vi "WPI_ADI_IMU_Open.vi"(8 "error in":errorcluster, 9 "AHRS Algorithm":enum16{"Complementary", "Madgwick"}(ring), 10 "Yaw Axis":enum16{"X", "Y", "Z"}(ring)=enum."Z", 11 "SPI Chip Select":T3=enum."SPI MXP") -> (0 "error out":errorcluster, 3 "ADI IMU Interrupt DevRef":T1={"SimpleGyroDevRef"={"DevStatus"={"status"=FALSE, "code"=0, "source"=""}, "Handle"=0, "SPI Bus"=enum."SPI On-Board, CS0", "Device Found"=FALSE, "Sample Rate"=0.0, "Device Ready"=FALSE, "Yaw Axis"=enum."Z", "AHRS Algorithm"=enum."Complementary"}, "InterruptRef"={"DevStatus"={"status"=FALSE, "code"=0, "source"=""}, "InterruptIndex"=enum."0"}} {"SimpleGyroDevRef"."Sample Rate" min=0.25 max=100.0 step=0.25})   [LabVIEW 2015, in "FRC ADI MXP IMU.lvlib"]
doc: "Initiates communication between an Analog Devices MXP IMU and the RoboRIO."
uses:
  FRC ADI MXP IMU.lvlib
  <vilib>/Rock Robotics/SystemInterfaces/spilib/spi_bus.ctl
  WPI_AnalogDevicesIMUInterruptDevRef.ctl
  WPI_AnalogDevicesIMUDevRef.ctl
  <vilib>/Rock Robotics/WPI/Interrupt/WPI_InterruptRef.ctl
  <vilib>/Rock Robotics/SystemInterfaces/Interrupt/FPGA_InterruptIndex.ctl
  <vilib>/Rock Robotics/WPI/SPI/WPI_SPIMode.ctl
  <vilib>/Rock Robotics/SystemInterfaces/DIO/FPGA_DIOChannel.ctl
  WPI_IMU_ADIS16448_Registers.ctl
  <vilib>/Rock Robotics/WPI/Counter/WPI_CounterDigitalInputToDigitalSource.vi
  <vilib>/Rock Robotics/SystemInterfaces/CounterEncoderSourceConvertion/FPGA_CounterEncoderSourceConvertionLVSourceTypeToFPGAType.vi
  <vilib>/Rock Robotics/WPI/Interrupt/WPI_InterruptCache.vi
  <vilib>/Rock Robotics/SystemInterfaces/Interrupt/FPGA_InterruptWriteConfiguration.vi
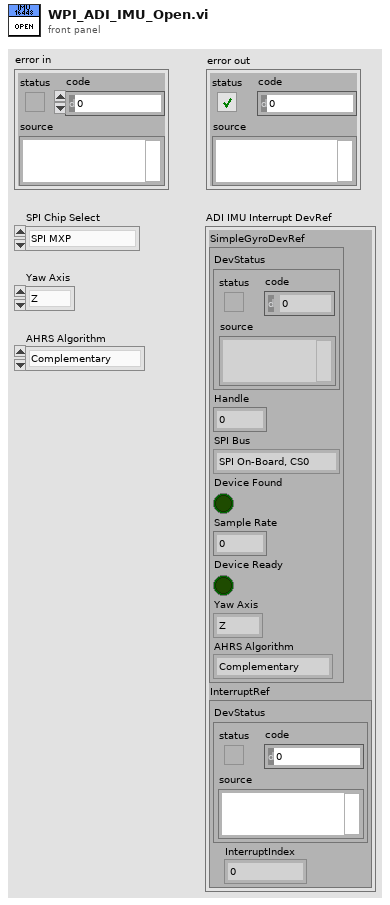
[diagram p1: front panel]
types:
  T1 = typedef "FRC ADI MXP IMU.lvlib/WPI_AnalogDevicesIMUInterruptDevRef.ctl" = cluster{"SimpleGyroDevRef":T2, "InterruptRef":T4}
  T2 = typedef "FRC ADI MXP IMU.lvlib/WPI_AnalogDevicesIMUDevRef.ctl" = cluster{"DevStatus":errorcluster, "Handle":i32, "SPI Bus":T3, "Device Found":bool, "Sample Rate":dbl, "Device Ready":bool, "Yaw Axis":enum16{"X", "Y", "Z"}, "AHRS Algorithm":enum16{"Complementary", "Madgwick"}}
  T3 = typedef "spi_bus.ctl" = enum16{"SPI On-Board, CS0", "SPI On-Board, CS1", "SPI On-Board, CS2", "SPI On-Board, CS3", "SPI MXP", "Invalid"}
  T4 = typedef "WPI_InterruptRef.ctl" = cluster{"DevStatus":errorcluster, "InterruptIndex":T5}
  T5 = typedef "FPGA_InterruptIndex.ctl" = enum8{"0", "1", "2", "3", "4", "5", "6", "7", "Invalid"}
  T6 = typedef "FPGA_DIOChannel.ctl" = enum8{"DIO 0", "DIO 1", "DIO 2", "DIO 3", "DIO 4", "DIO 5", "DIO 6", "DIO 7", "DIO 8", "DIO 9", "DIO MXP 0", "DIO MXP 1", "DIO MXP 2", "DIO MXP 3", "DIO MXP 4", "DIO MXP 5", "DIO MXP 6", "DIO MXP 7", "DIO MXP 8", "DIO MXP 9", "DIO MXP 10", "DIO MXP 11", "DIO MXP 12", "DIO MXP 13", "DIO MXP 14", "DIO MXP 15", "Invalid"}
  T7 = typedef "WPI_SPIMode.ctl" = enum16{"Mode 0 (Clk Idle Low,Sample on Leading)", "Mode 1 (Clk Idle Low,Sample on Trailing)", "Mode 2 (Clk Idle High,Sample on Leading)", "Mode 3 (Clk Idle High,Sample on Trailing)"}
  T8 = typedef "FRC ADI MXP IMU.lvlib/WPI_IMU_ADIS16448_Registers.ctl" = u8
  T9 = typedef "WPI_DigitalOutputDevRef.ctl" = cluster{"DIO Channel":T6, "DevStatus":errorcluster}
  T10 = typedef "WPI_SPIDevRef.ctl" = cluster{"DevStatus":errorcluster, "Handle":i32, "SPI Bus":T3}
  T11 = typedef "WPI_DigitalInputDevRef.ctl" = cluster{"DevStatus":errorcluster, "DIO Channel":T6}
  T12 = typedef "FPGA_CounterEncoderSourceConvertionLVSourceType.ctl" = cluster{"DevStatus":errorcluster, "AnalogTriggerMode?":bool, "DigitalMode":cluster{"DIO Channel":T13}, "AnalogTriggerMode":cluster{"AnalogTriggerIndex":T14, "OutputType":T15}}
  T13 = typedef "FPGA_DIODigitalSourceChannel.ctl" = enum8{"DIO 0", "DIO 1", "DIO 2", "DIO 3", "DIO 4", "DIO 5", "DIO 6", "DIO 7", "DIO 8", "DIO 9", "DIO MXP 0", "DIO MXP 1", "DIO MXP 2", "DIO MXP 3", "DIO MXP 4", "DIO MXP 5", "DIO MXP 6", "DIO MXP 7", "DIO MXP 8", "DIO MXP 9", "DIO MXP 10", "DIO MXP 11", "DIO MXP 12", "DIO MXP 13", "DIO MXP 14", "DIO MXP 15", "Disabled"}
  T14 = typedef "FPGA_AnalogTriggerIndex.ctl" = enum8{"Trig 0", "Trig 1", "Trig 2", "Trig 3", "Trig 4", "Trig 5", "Trig 6", "Trig 7", "Invalid"}
  T15 = typedef "FPGA_AnalogTriggerOutType.ctl" = enum16{"InWindow", "TriggerState", "Rising", "Falling"}
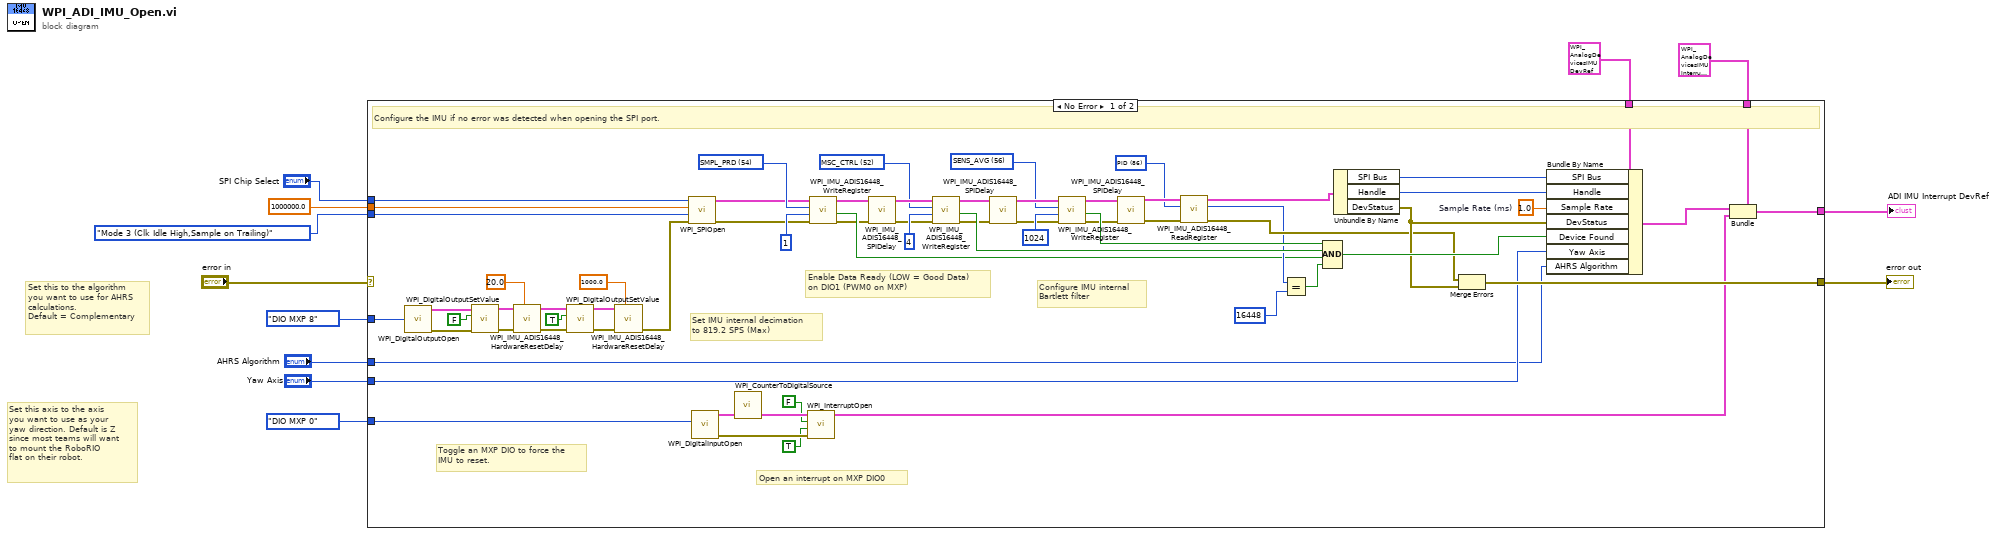
[diagram p0: block diagram]
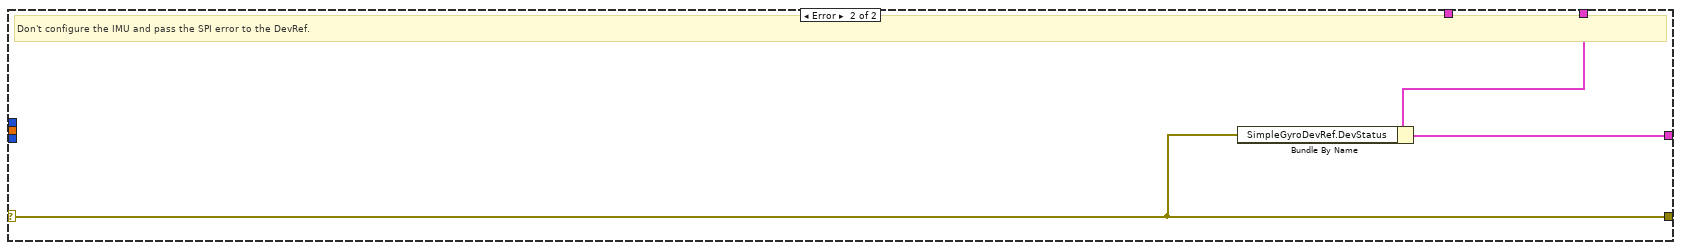
[diagram p2: hidden frame]
diagram:
  # "Set this to the algorithm\nyou want to use for AHRS\ncalculations. \nDefault = Complementary"
  # "Set this axis to the axis\nyou want to use as your\nyaw direction. Default is Z\nsince most teams will want \nto mount the RoboRIO\nflat on their robot."
  n1 = case shown="No Error" "error in" {
    selector: "error in" -> [_ w79]
    tunnel: "SPI Chip Select" -> [w77 _]
    tunnel: 1000000.0 ("Clock Rate (Hz)") -> [w76 _]
    tunnel: WPI_SPIMode."Mode 3 (Clk Idle High,Sample on Trailing)" ("Mode (3)") -> [w75 _]
    tunnel: [w66 w79] -> w8
    tunnel: T2 {"DevStatus"={"status"=FALSE, "code"=0, "source"=""}, "Handle"=0, "SPI Bus"=enum."SPI On-Board, CS0", "Device Found"=FALSE, "Sample Rate"=0.0, "Device Ready"=FALSE, "Yaw Axis"=enum."Z", "AHRS Algorithm"=enum."Complementary"} ("SimpleGyroDevRef 2") -> [w74 _]
    tunnel: [w56 w78] -> w1
    tunnel: T1 {"SimpleGyroDevRef"={"DevStatus"={"status"=FALSE, "code"=0, "source"=""}, "Handle"=0, "SPI Bus"=enum."SPI On-Board, CS0", "Device Found"=FALSE, "Sample Rate"=0.0, "Device Ready"=FALSE, "Yaw Axis"=enum."Z", "AHRS Algorithm"=enum."Complementary"}, "InterruptRef"={"DevStatus"={"status"=FALSE, "code"=0, "source"=""}, "InterruptIndex"=enum."0"}} ("output cluster") -> [w55 w80]
    tunnel: FPGA_DIOChannel."DIO MXP 0" ("DIO Channel") -> [w54 _]
    tunnel: "Yaw Axis" -> [w47 _]
    tunnel: "AHRS Algorithm" -> [w46 _]
    tunnel: FPGA_DIOChannel."DIO MXP 8" ("DIO Channel") -> [w16 _]
    frame No Error {
      w30 = T8 54 items=["GLOB_CMD"=62, "SEQ_CNT"=58, "SMPL_PRD"=54, "SENS_AVG"=56, "MSC_CTRL"=52, "ERROR_FLAGS"=60, "TEMP"=44, "BARO"=40, "Z_MAG"=36, "Y_MAG"=32, "X_MAG"=28, "Z_ACCEL"=24, "Y_ACCEL"=20, "X_ACCEL"=16, "Z_GYRO"=12, "Y_GYRO"=8, "X_GYRO"=4, "PID"=86] ("ADIS16448 Register")
      w31 = T8 52 items=["GLOB_CMD"=62, "SEQ_CNT"=58, "SMPL_PRD"=54, "SENS_AVG"=56, "MSC_CTRL"=52, "ERROR_FLAGS"=60, "TEMP"=44, "BARO"=40, "Z_MAG"=36, "Y_MAG"=32, "X_MAG"=28, "Z_ACCEL"=24, "Y_ACCEL"=20, "X_ACCEL"=16, "Z_GYRO"=12, "Y_GYRO"=8, "X_GYRO"=4, "PID"=86] ("ADIS16448 Register")
      w32 = T8 56 items=["GLOB_CMD"=62, "SEQ_CNT"=58, "SMPL_PRD"=54, "SENS_AVG"=56, "MSC_CTRL"=52, "ERROR_FLAGS"=60, "TEMP"=44, "BARO"=40, "Z_MAG"=36, "Y_MAG"=32, "X_MAG"=28, "Z_ACCEL"=24, "Y_ACCEL"=20, "X_ACCEL"=16, "Z_GYRO"=12, "Y_GYRO"=8, "X_GYRO"=4, "PID"=86] ("ADIS16448 Register")
      w33 = T8 86 items=["GLOB_CMD"=62, "SEQ_CNT"=58, "SMPL_PRD"=54, "SENS_AVG"=56, "MSC_CTRL"=52, "ERROR_FLAGS"=60, "TEMP"=44, "BARO"=40, "Z_MAG"=36, "Y_MAG"=32, "X_MAG"=28, "Z_ACCEL"=24, "Y_ACCEL"=20, "X_ACCEL"=16, "Z_GYRO"=12, "Y_GYRO"=8, "X_GYRO"=4, "PID"=86] ("ADIS16448 Register")
      w71 = 1.0  # Sample Rate (ms)
      # "Toggle an MXP DIO to force the\nIMU to reset."
      # "Open an interrupt on MXP DIO0"
      # "Configure IMU internal\nBartlett filter"
      # "Enable Data Ready (LOW = Good Data) \non DIO1 (PWM0 on MXP)"
      # "Set IMU internal decimation\nto 819.2 SPS (Max)"
      # "Configure the IMU if no error was detected when opening the SPI port."
      n2 = call <vilib>:"WPI_DigitalOutputOpen.vi"("DIO Channel"=w16) -> ("error out"=w26:errorcluster, "DigitalOutputDevRef"=w27:T9)  [unwired: 9 in]
      n3 = call <vilib>:"WPI_DigitalOutputSetValue.vi"("error in (no error)"=w26, "Value"=FALSE, "DigitalOutputDevRef"=w27) -> ("error out"=w24:errorcluster, "DigitalOutputDevRef"=w25:T9)  [unwired: 7 in]
      n4 = call "WPI_IMU_ADIS16448_HardwareResetDelay.vi"("Delay (ms)"=20.0, "error in"=w24, "DigitalOutputDevRef"=w25) -> ("error out"=w23:errorcluster, "DigitalOutputDevRef"=w22:T9)  [unwired: 7 in]
      n5 = call <vilib>:"WPI_DigitalOutputSetValue.vi"("error in (no error)"=w23, "Value"=TRUE, "DigitalOutputDevRef"=w22) -> ("error out"=w20:errorcluster, "DigitalOutputDevRef"=w19:T9)  [unwired: 7 in]
      n6 = call "WPI_IMU_ADIS16448_HardwareResetDelay.vi"("Delay (ms)"=1000.0, "error in"=w20, "DigitalOutputDevRef"=w19) -> ("error out"=w15:errorcluster)  [unwired: 7 in, 1 out]
      n7 = call <vilib>:"WPI_SPIOpen.vi"("error in"=w15, "Mode (3)"=w75, "Clock Rate (Hz)"=w76, "SPI Bus"=w77) -> ("error out"=w13:errorcluster, "SPIDevRef"=w14:T10)  [unwired: 6 in]
      n8 = call <vilib>:"WPI_DigitalInputOpen.vi"("DIO Channel"=w54) -> ("error out"=w61:errorcluster, "DigitalInputDevRef"=w63:T11)  [unwired: 9 in]
      n9 = call-poly <vilib>:"WPI_CounterToDigitalSource.vi"("DigitalInputDevRef"=w63) -> ("Digital Source"=w62:T12)  [unwired: 6 in]
      n10 = call <vilib>:"WPI_InterruptOpen.vi"("error in (no error)"=w61, "Falling Edge"=TRUE, "Rising Edge"=FALSE, "Source"=w62) -> ("InterruptRef"=w58:T4)  [unwired: 6 in, 1 out]
      n11 = call "WPI_IMU_ADIS16448_WriteRegister.vi"("error in (no error)"=w13, "Data"=u16 1, "ADIS16448 Register"=w30, "SPIDevRef in"=w14) -> ("error out"=w44:errorcluster, "Write OK?"=w48:bool, "SPIDevRef out"=w45:T10)  [unwired: 4 in, 1 out]
      n12 = call "WPI_IMU_ADIS16448_SPIDelay.vi"("error in"=w44, "SPIDevRef in"=w45) -> ("error out"=w42:errorcluster, "SPIDevRef out"=w43:T10)  [unwired: 8 in]
      n13 = call "WPI_IMU_ADIS16448_WriteRegister.vi"("error in (no error)"=w42, "Data"=u16 4, "ADIS16448 Register"=w31, "SPIDevRef in"=w43) -> ("error out"=w40:errorcluster, "Write OK?"=w68:bool, "SPIDevRef out"=w41:T10)  [unwired: 4 in, 1 out]
      n14 = call "WPI_IMU_ADIS16448_SPIDelay.vi"("error in"=w40, "SPIDevRef in"=w41) -> ("error out"=w39:errorcluster, "SPIDevRef out"=w38:T10)  [unwired: 8 in]
      n15 = call "WPI_IMU_ADIS16448_WriteRegister.vi"("error in (no error)"=w39, "Data"=u16 1024, "ADIS16448 Register"=w32, "SPIDevRef in"=w38) -> ("error out"=w36:errorcluster, "Write OK?"=w64:bool, "SPIDevRef out"=w37:T10)  [unwired: 4 in, 1 out]
      n16 = call "WPI_IMU_ADIS16448_SPIDelay.vi"("error in"=w36, "SPIDevRef in"=w37) -> ("error out"=w34:errorcluster, "SPIDevRef out"=w35:T10)  [unwired: 8 in]
      n17 = call "WPI_IMU_ADIS16448_ReadRegister.vi"("error in (no error)"=w34, "ADIS16448 Register"=w33, "SPIDevRef in"=w35) -> ("error out"=w52:errorcluster, "Register Value"=w51:u16, "SPIDevRef out"=w53:T10)  [unwired: 6 in]
      n18 = Equal?(x=w51, y=u16 16448) -> (x = y?=w29:bool)
      n19 = Compound Arithmetic op=AND(w64, w68, w48, w29) -> (w69:bool)
      n20 = Unbundle By Name(w53) -> ("SPI Bus"=w73:T3, "Handle"=w72:i32, "DevStatus"=w67:errorcluster)
      n21 = Merge Errors(w52, w67) -> (w66:errorcluster)
      n22 = Bundle By Name(cluster=w74, "SPI Bus"=w73, "Handle"=w72, "Sample Rate"=w71, "DevStatus"=w67, "Device Found"=w69, "Yaw Axis"=w47, "AHRS Algorithm"=w46) -> (w57:T2)
      n23 = Bundle(cluster=w55, "SimpleGyroDevRef"=w57, "InterruptRef"=w58) -> (w56:T1)
    }
    frame Error {
      # "Don't configure the IMU and pass the SPI error to the DevRef."
      n24 = Bundle By Name(cluster=w80, "SimpleGyroDevRef.DevStatus"=w79) -> (w78:T1)
    }
  }
  "error out" <- w8
  "ADI IMU Interrupt DevRef" <- w1
